vi "Update.vi"(8 "error in (no error)":errorcluster, 11 "TileTimer in":refnum<class "TileTimer.lvclass">) -> (0 "error out":errorcluster, 3 "TileTimer out":refnum<class "TileTimer.lvclass">)   [LabVIEW 2019, in "RT_Game.lvlib" / "TileTimer.lvclass"]
uses:
  TileTimer.lvclass
  TileTimer.lvclass/TileTimer.ctl
  GameObject/GameObject.lvclass
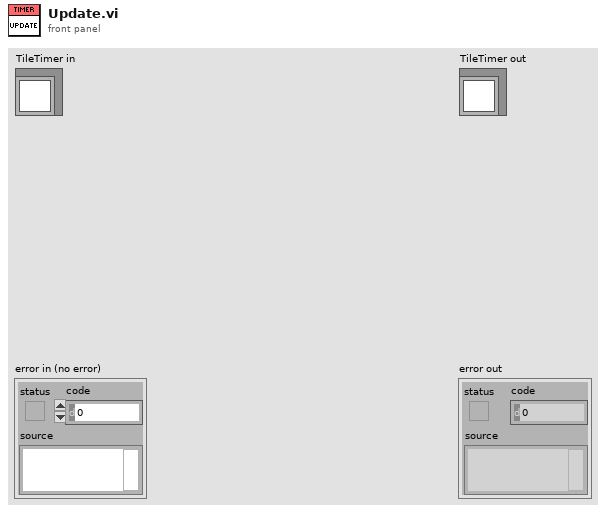
[diagram p1: front panel]
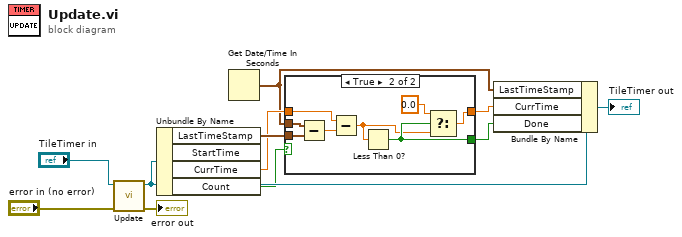
[diagram p0: block diagram]
diagram:
  n1 = call-parent "Update.vi"("error in (no error)"="error in (no error)", "GameObject in"="TileTimer in") -> ("error out"=→"error out":errorcluster, "GameObject out"=w8:refnum<class "TileTimer.lvclass">)  [unwired: 8 in]
  n2 = Unbundle By Name(w8) -> ("LastTimeStamp"=w7:timestamp, "CurrTime"=w3:dbl, "Count"=w1:bool)  [unwired: 1 out]
  n3 = Get Date/Time In Seconds() -> (seconds since 1Jan1904=w2:timestamp)
  n4 = case shown="True" w1 {
    tunnel: w7 -> [_ w20]
    tunnel: [w12 w19] -> w5
    tunnel: [_ w18] -> w4
    tunnel: w3 -> [w12 w16]
    tunnel: w2 -> [_ w13]
    frame False {
    }
    frame True {
      n5 = Subtract(x=w13, y=w20) -> (x-y=w15:dbl)
      n6 = Subtract(x=w16, y=w15) -> (x-y=w14:dbl)
      n7 = Less Than 0?(x=w14) -> (x < 0?=w18:bool)
      n8 = Select(t=0.0, s=w18, f=w14) -> (s? t:f=w19:dbl)
    }
  }
  n9 = Bundle By Name(cluster=w8, "LastTimeStamp"=w2, "CurrTime"=w5, "Done"=w4) -> (→"TileTimer out":refnum<class "TileTimer.lvclass">)
